vi "MS SQL_InRFID_STN70.vi"(6 "RFID":string, 7 "OP70_ASR":T1, 8 "error in (no error)":errorcluster, 11 "Ref in":T2={"MS SQL Connection"=refnum, "UDL File"=path "", "Time"="", "DCODE"="", "WIP+1"=0, "MC No?"=0, "POKAYOKE?"=FALSE, "Expected Result"="", "Result [Status]"="", "Clock"=0.0, "RFID"="", "WIP Queue"=refnum, "TS Parameter"={"ProfitCenterCode"="", "LineCode"="", "WorkOrderNumber"="", "Model"="", "Model_with_Prefix"="", "VendorCode"="", "SetParameterDateCode"="", "PokaYoke"=0, "Target"=1, "Live_DateCode"="", "CustomerPartNumber"="", "Hand"="", "Ent_Stamp"=timestamp(0 s since 1904-01-01), "STS_CD"=0.0}, "Data_Queue"=[], "RFID Serial No."=""} {"TS Parameter"."Target" min=1 max=100000; "TS Parameter"."PokaYoke" min=0 max=1}) -> (0 "error out":errorcluster, 1 "Message":picture, 3 "Ref Out":T2={"MS SQL Connection"=refnum, "UDL File"=path "", "Time"="", "DCODE"="", "WIP+1"=0, "MC No?"=0, "POKAYOKE?"=FALSE, "Expected Result"="", "Result [Status]"="", "Clock"=0.0, "RFID"="", "WIP Queue"=refnum, "TS Parameter"={"ProfitCenterCode"="", "LineCode"="", "WorkOrderNumber"="", "Model"="", "Model_with_Prefix"="", "VendorCode"="", "SetParameterDateCode"="", "PokaYoke"=0, "Target"=1, "Live_DateCode"="", "CustomerPartNumber"="", "Hand"="", "Ent_Stamp"=timestamp(0 s since 1904-01-01), "STS_CD"=0.0}, "Data_Queue"=[], "RFID Serial No."=""} {"TS Parameter"."Target" min=1 max=100000; "TS Parameter"."PokaYoke" min=0 max=1})   [LabVIEW 2020]
uses:
  Controls/TD SQL.ctl
  <vilib>/addons/database/Connection.llb/Conn ObjectReference.ctl
  Controls/WIP_State.ctl
  Controls/TS_Parameter.ctl
  <vilib>/addons/database/NI_Database_API.lvlib
panel:
  in  "[CT]":dbl
  in  "[ASR_DISTANCE_ACTUAL]":dbl
  in  "[ASR_DISTANCE_SET]":dbl
  in  "[ASR_LOAD_MAX]":dbl
  in  "[ASR_LOAD_ACTUAL]":dbl
  out "resulting string":string
  # "OP80"
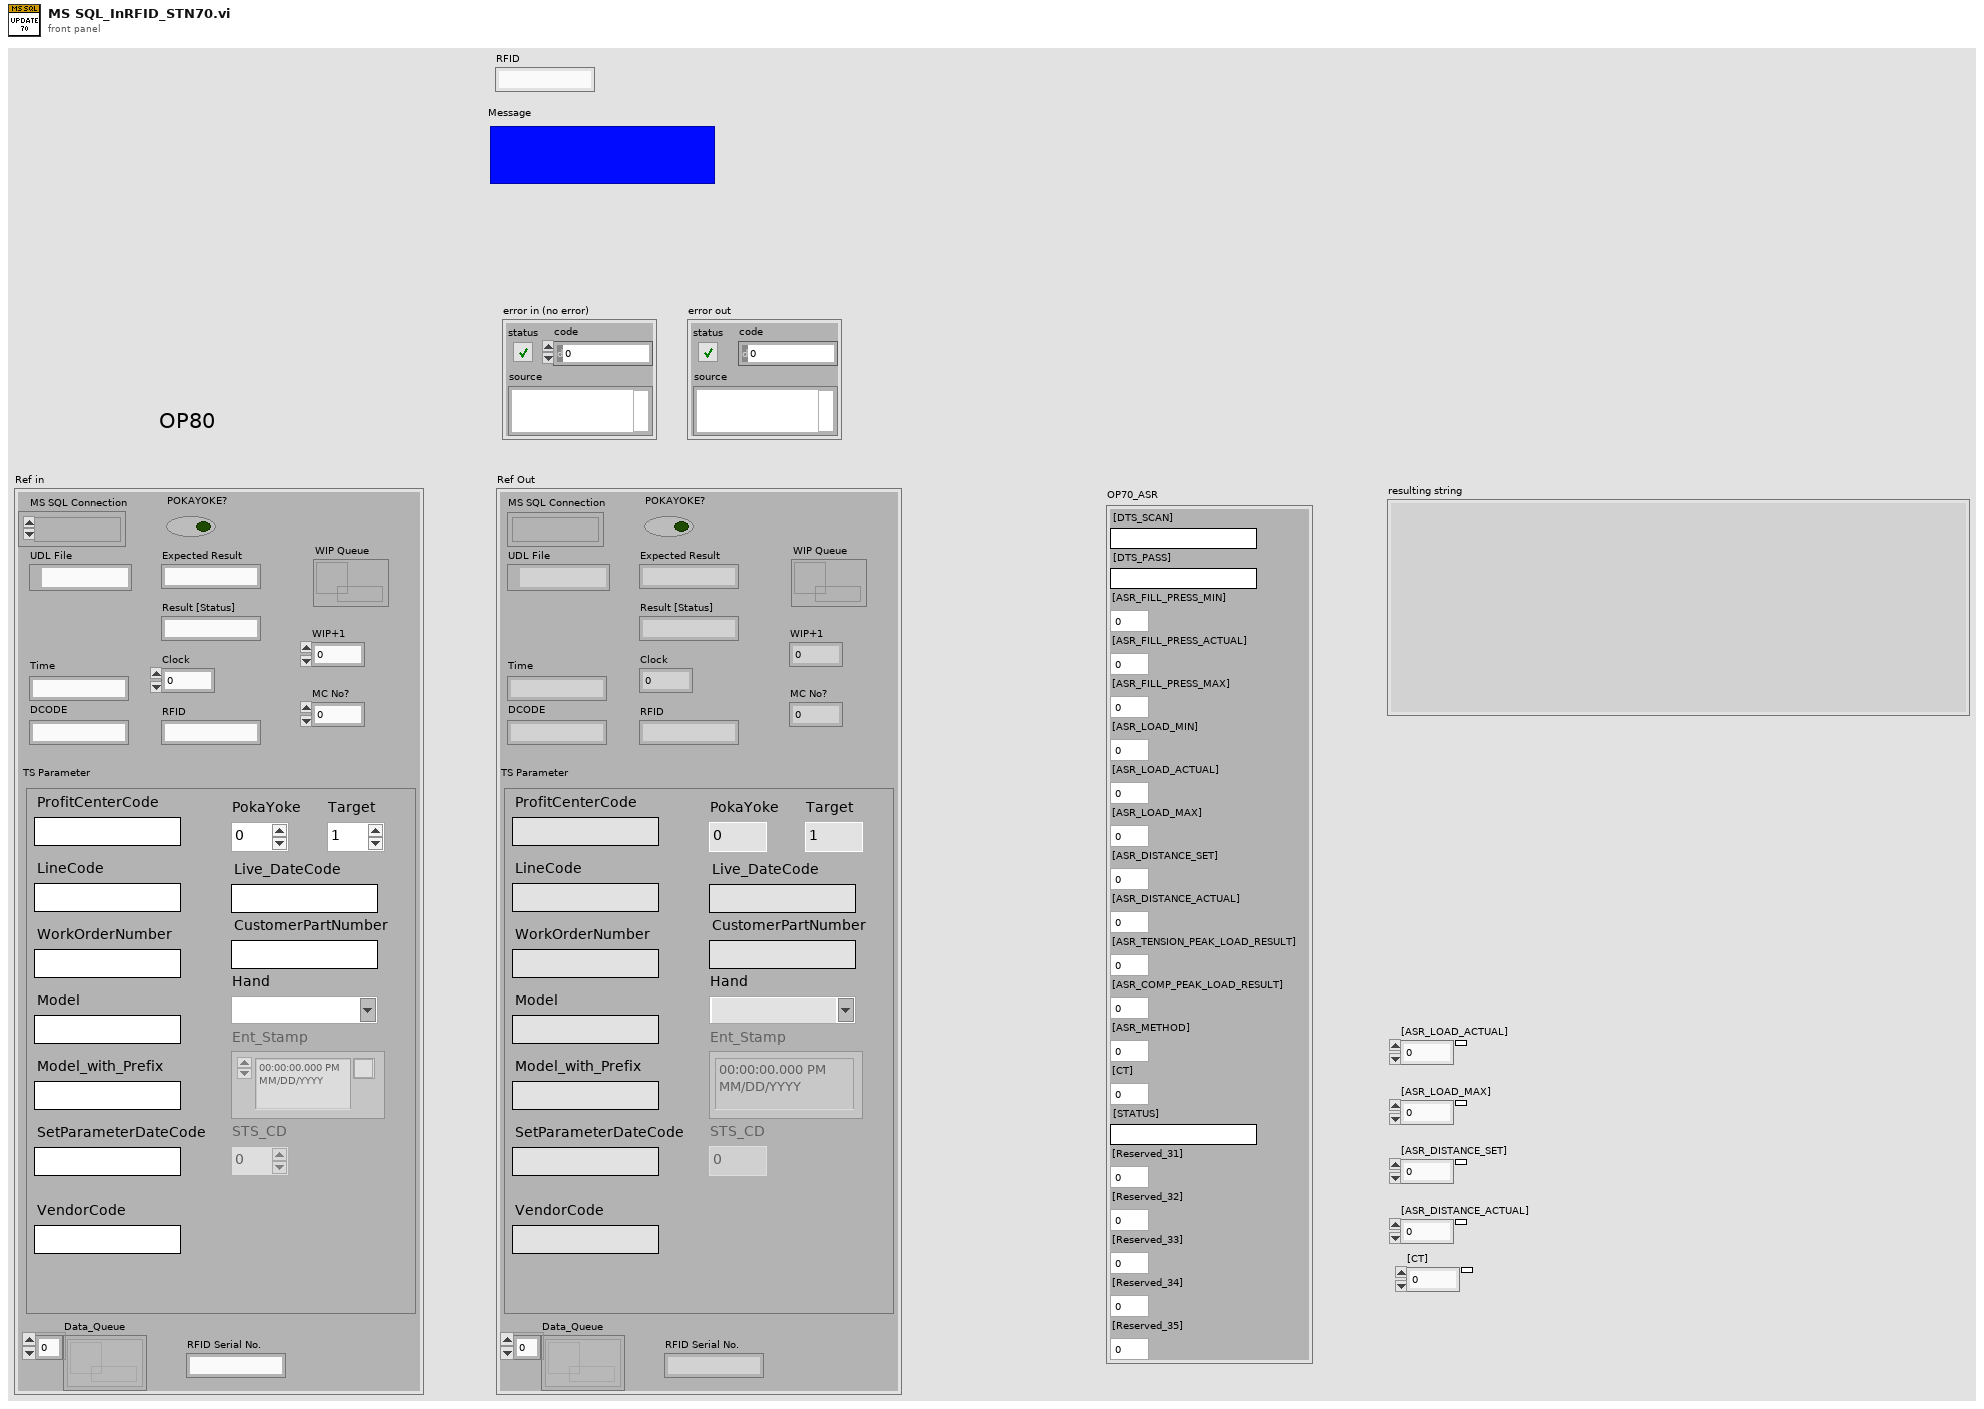
[diagram p1: front panel]
types:
  T1 = cluster{"[DTS_SCAN]":string, "[DTS_PASS]":string, "[ASR_FILL_PRESS_MIN]":dbl, "[ASR_FILL_PRESS_ACTUAL]":dbl, "[ASR_FILL_PRESS_MAX]":dbl, "[ASR_LOAD_MIN]":dbl, "[ASR_LOAD_ACTUAL]":dbl, "[ASR_LOAD_MAX]":dbl, "[ASR_DISTANCE_SET]":dbl, "[ASR_DISTANCE_ACTUAL]":dbl, "[ASR_TENSION_PEAK_LOAD_RESULT]":dbl, "[ASR_COMP_PEAK_LOAD_RESULT]":dbl, "[ASR_METHOD]":dbl, "[CT]":dbl, "[STATUS]":string, "[Reserved_31]":dbl, "[Reserved_32]":dbl, "[Reserved_33]":dbl, "[Reserved_34]":dbl, "[Reserved_35]":dbl}
  T2 = typedef "TD SQL.ctl" = cluster{"MS SQL Connection":T3, "UDL File":path, "Time":string, "DCODE":string, "WIP+1":i64, "MC No?":i32, "POKAYOKE?":bool, "Expected Result":string, "Result [Status]":string, "Clock":dbl, "RFID":string, "WIP Queue":refnum<queue>, "TS Parameter":T4, "Data_Queue":refnum<queue>[], "RFID Serial No.":string}
  T3 = typedef "NI_Database_API.lvlib/Conn ObjectReference.ctl" = refnum<k1>
  T4 = typedef "TS_Parameter.ctl" = cluster{"ProfitCenterCode":string, "LineCode":string, "WorkOrderNumber":string, "Model":string, "Model_with_Prefix":string, "VendorCode":string, "SetParameterDateCode":string, "PokaYoke":i32, "Target":i32, "Live_DateCode":string, "CustomerPartNumber":string, "Hand":string, "Ent_Stamp":timestamp, "STS_CD":dbl}
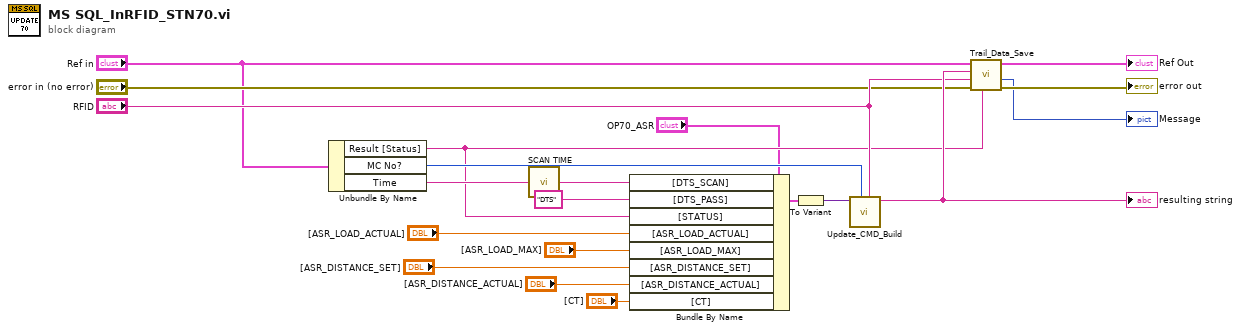
[diagram p0: block diagram]
diagram:
  n1 = Unbundle By Name("Ref in") -> ("Result [Status]"=w8:string, "MC No?"=w9:i32, "Time"=w10:string)
  n2 = call "SCAN TIME.vi"("Time in"=w10) -> ("Time out"=w17:string)
  n3 = Bundle By Name(cluster="OP70_ASR", "[DTS_SCAN]"=w17, "[DTS_PASS]"="DTS", "[STATUS]"=w8, "[ASR_LOAD_ACTUAL]"="[ASR_LOAD_ACTUAL]", "[ASR_LOAD_MAX]"="[ASR_LOAD_MAX]", "[ASR_DISTANCE_SET]"="[ASR_DISTANCE_SET]", "[ASR_DISTANCE_ACTUAL]"="[ASR_DISTANCE_ACTUAL]", "[CT]"="[CT]") -> (w18:T1)
  n4 = To Variant(anything=w18) -> (Variant=w20:variant)
  n5 = call "Update_CMD_Build.vi"("RFID"="RFID", "Machine No"=w9, "Variant"=w20) -> ("Update Query"=w15:string)  [unwired: 5 in, 1 out]
  "resulting string" <- w15
  n6 = call "Trail_Data_Save.vi"("Status"=w8, "error in (no error)"="error in (no error)", "RFID"="RFID", "Query"=w15, "Ref in"="Ref in") -> ("error out"=→"error out":errorcluster, "Message"=→"Message":picture, "Ref Out"=→"Ref Out":T2)  [unwired: 1 in, 1 out]
